vi "Reference_Inst_Info_2_string.vi"(1 "Reference instrument":T2={"high limit (10V)"=4.0, "low limit (-10V)"=0.0, "Ch No"=4, "Off ch no"=0, "Calib filename"=path "", "Ref Instrument type"=enum."Enter Value"} {"Off ch no" min=0 max=1; "Ch No" min=0 max=50; "low limit (-10V)" min=-10 max=10 format="%.1f"; "high limit (10V)" min=-10 max=10 format="%.1f"}, 2 "Reference Name":string="Instrument to calibrate") -> (0 "Setup String":string)   [LabVIEW 2013]
uses:
  Controls/Ref_Inst_type.ctl
  Calib_setup.ctl
panel:
  in  "Ref Instrument type":T1=enum."LDA"
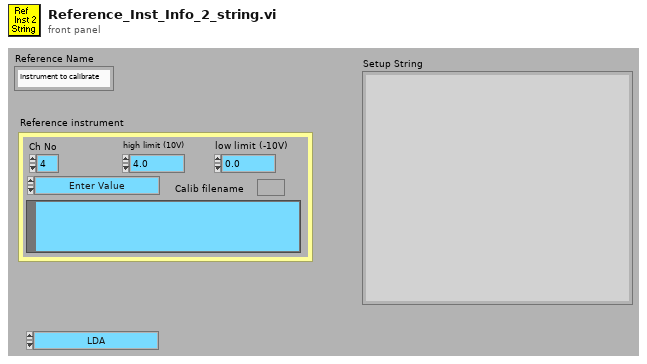
[diagram p1: front panel]
types:
  T1 = typedef "Ref_Inst_type.ctl" = enum16{"Propellor anemometer", "Pressure Transducer", "Raw voltage", "Pitot-static tube", "Preston tube", "Generic Linear", "Generic Polynomial", "Thermocouple", "LDA", "Enter Value", "ADAM Channel"}
  T2 = typedef "Calib_setup.ctl" = cluster{"high limit (10V)":sgl, "low limit (-10V)":sgl, "Ch No":i16, "Off ch no":i8, "Calib filename":path, "Ref Instrument type":T1}
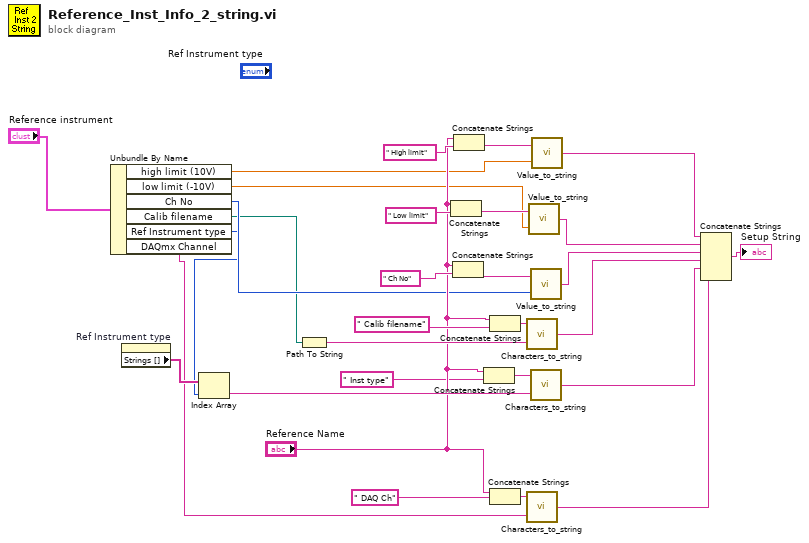
[diagram p0: block diagram]
diagram:
  n1 = Unbundle By Name("Reference instrument") -> ("high limit (10V)"=w9:sgl, "low limit (-10V)"=w8:sgl, "Ch No"=w7:i16, "Calib filename"=w6:path, "Ref Instrument type"=w5:T1, "DAQmx Channel"=w4:tag)
  n2 = property on="Ref Instrument type" class="Enum (strict)"() -> ("Strings []"=w21:string[])  [unwired: 2 in, 2 out]
  n3 = Index Array(array=w21, index=w5) -> (element=w20:string)
  n4 = Path To String(path=w6) -> (string=w24:string)
  n5 = Concatenate Strings("Reference Name", " Low limit") -> (w27:string)
  n6 = Concatenate Strings("Reference Name", " Ch No") -> (w28:string)
  n7 = Concatenate Strings("Reference Name", " High limit") -> (w26:string)
  n8 = Concatenate Strings("Reference Name", " Inst type") -> (w17:string)
  n9 = Concatenate Strings("Reference Name", " Calib filename") -> (w23:string)
  n10 = Concatenate Strings("Reference Name", " DAQ Ch") -> (w2:string)
  n11 = call "Characters_to_string.vi"("Characters to write"=w24, "Label for characters"=w23) -> ("Output string"=w14:string)
  n12 = call "Characters_to_string.vi"("Characters to write"=w4, "Label for characters"=w2) -> ("Output string"=w10:string)
  n13 = call "Value_to_string.vi"("Value"=w8, "Label for value"=w27) -> ("Output string"=w11:string)  [unwired: 1 in]
  n14 = call "Value_to_string.vi"("Value"=w7, "Label for value"=w28) -> ("Output string"=w12:string)  [unwired: 1 in]
  n15 = call "Characters_to_string.vi"("Characters to write"=w20, "Label for characters"=w17) -> ("Output string"=w15:string)
  n16 = call "Value_to_string.vi"("Value"=w9, "Label for value"=w26) -> ("Output string"=w13:string)  [unwired: 1 in]
  n17 = Concatenate Strings(w13, w11, w12, w14, w15, w10) -> (→"Setup String":string)
